vi "CANOpen_SDO Update status channels Dyn Read.vi"(8 "error in (no error)":errorcluster, 9 "Status Data":T2, 10 "Chan Refs":T1[](array[typedef]) format="%.0x", 11 "index of element":i32) -> (0 "error out":errorcluster)   [LabVIEW 2013, in "CANOpen Addon Custom Device.lvlib"]
uses:
  CANOpen Addon Custom Device.lvlib
  Async VIs/CANOpen_Main/SubVIs/CanOpen_SDO Dynamic queue.ctl
  Shared Code/CANOpen_SDO queue W data.ctl
  Shared Code/CANOpen_SDO queue mode.ctl
  Shared Code/CANOpen_PDO Data Type in queue.ctl
  <vilib>/NI Veristand/Custom Device API/Data Reference.ctl
  <vilib>/NI Veristand/Custom Device API/Global Data Refs.vi
  <vilib>/NI Veristand/Custom Device API/Custom Device API.lvlib
  Debug/SubVIs/Global debug.vi
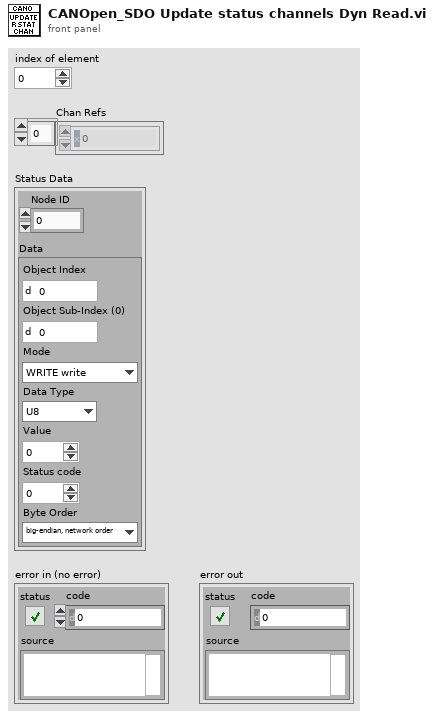
[diagram p1: front panel]
types:
  T1 = typedef "Custom Device API.lvlib/Data Reference.ctl" = i32
  T2 = typedef "CANOpen Addon Custom Device.lvlib/CanOpen_SDO Dynamic queue.ctl" = cluster{"Node ID":u8, "Data":T3}
  T3 = typedef "CANOpen Addon Custom Device.lvlib/CANOpen_SDO queue W data.ctl" = cluster{"Object Index":u16, "Object Sub-Index (0)":u8, "Mode":T4, "Data Type":T5, "Value":dbl, "Status code":dbl, "Byte Order":enum16{"big-endian, network order", "little-endian"}}
  T4 = typedef "CANOpen Addon Custom Device.lvlib/CANOpen_SDO queue mode.ctl" = enum16{"WRITE write", "WRITE response", "READ write", "READ response"}
  T5 = typedef "CANOpen Addon Custom Device.lvlib/CANOpen_PDO Data Type in queue.ctl" = enum16{"U8", "U16", "U32", "I8", "I16", "I32", "Single", "Double"}
  T6 = enum16{"big-endian, network order", "little-endian"}
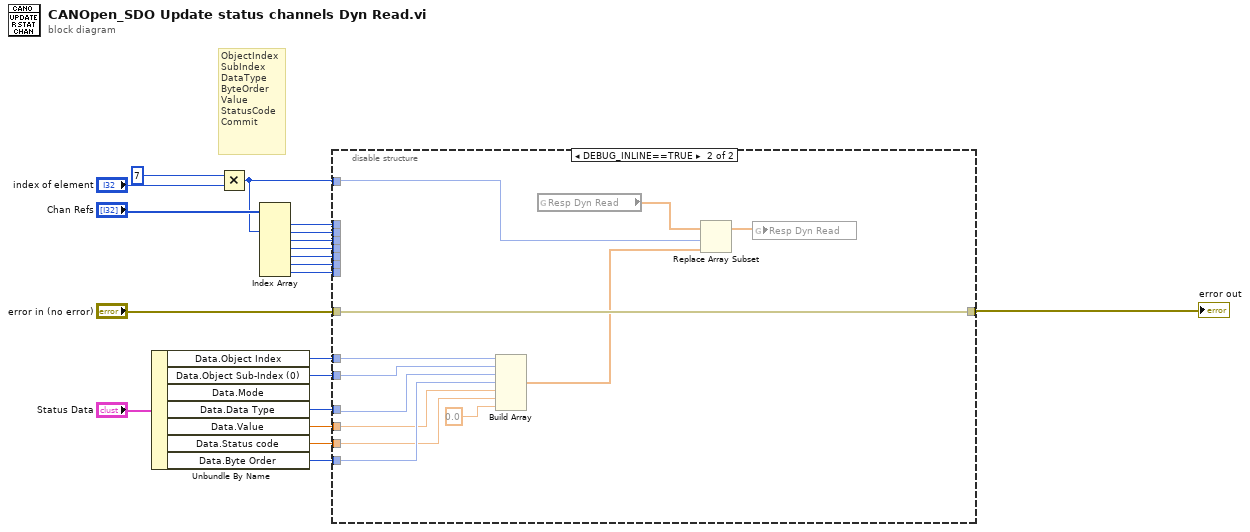
[diagram p0: block diagram]
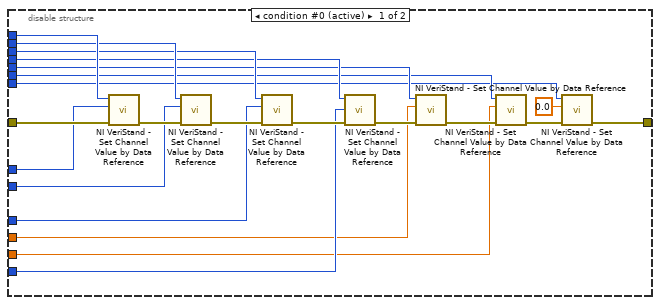
[diagram p2: hidden frame]
diagram:
  # "ObjectIndex\nSubIndex\nDataType\nByteOrder\nValue\nStatusCode\nCommit"
  n1 = Unbundle By Name("Status Data") -> ("Data.Object Index"=w7:u16, "Data.Object Sub-Index (0)"=w6:u8, "Data.Data Type"=w5:T5, "Data.Value"=w3:dbl, "Data.Status code"=w2:dbl, "Data.Byte Order"=w4:T6)  [unwired: 1 out]
  n2 = Multiply(x=7, y="index of element") -> (x*y=w1:i32)
  n3 = Index Array(array="Chan Refs", index #1=w1) -> (element #1=w14:T1, element #2=w13:T1, element #3=w12:T1, element #4=w11:T1, element #5=w10:T1, element #6=w9:T1, element #7=w8:T1)  [unwired: 6 in]
  n4 = disable-structure shown="DEBUG_INLINE==TRUE" {
    disable-tunnel: "error in (no error)" -> [w42 w54]
    disable-tunnel: [w35 w54] -> w20
    disable-tunnel: w14 -> [w34 _]
    disable-tunnel: w13 -> [w33 _]
    disable-tunnel: w12 -> [w32 _]
    disable-tunnel: w11 -> [w31 _]
    disable-tunnel: w10 -> [w30 _]
    disable-tunnel: w9 -> [w29 _]
    disable-tunnel: w8 -> [w28 _]
    disable-tunnel: w7 -> [w27 w53]
    disable-tunnel: w6 -> [w26 w52]
    disable-tunnel: w5 -> [w25 w51]
    disable-tunnel: w4 -> [w24 w46]
    disable-tunnel: w3 -> [w23 w45]
    disable-tunnel: w2 -> [w22 w44]
    disable-tunnel: w1 -> [_ w50]
    frame condition #0 (active) {
      n5 = call <vilib>:"NI VeriStand - Set Channel Value by Data Reference.vi"("error in (no error)"=w42, "Value"=w27, "Data Reference in"=w34) -> ("error out"=w41:errorcluster)  [unwired: 8 in]
      n6 = call <vilib>:"NI VeriStand - Set Channel Value by Data Reference.vi"("error in (no error)"=w41, "Value"=w26, "Data Reference in"=w33) -> ("error out"=w40:errorcluster)  [unwired: 8 in]
      n7 = call <vilib>:"NI VeriStand - Set Channel Value by Data Reference.vi"("error in (no error)"=w40, "Value"=w25, "Data Reference in"=w32) -> ("error out"=w39:errorcluster)  [unwired: 8 in]
      n8 = call <vilib>:"NI VeriStand - Set Channel Value by Data Reference.vi"("error in (no error)"=w39, "Value"=w24, "Data Reference in"=w31) -> ("error out"=w38:errorcluster)  [unwired: 8 in]
      n9 = call <vilib>:"NI VeriStand - Set Channel Value by Data Reference.vi"("error in (no error)"=w38, "Value"=w23, "Data Reference in"=w30) -> ("error out"=w37:errorcluster)  [unwired: 8 in]
      n10 = call <vilib>:"NI VeriStand - Set Channel Value by Data Reference.vi"("error in (no error)"=w37, "Value"=w22, "Data Reference in"=w29) -> ("error out"=w36:errorcluster)  [unwired: 8 in]
      n11 = call <vilib>:"NI VeriStand - Set Channel Value by Data Reference.vi"("error in (no error)"=w36, "Value"=0.0, "Data Reference in"=w28) -> ("error out"=w35:errorcluster)  [unwired: 8 in]
    }
    frame condition #1 {
      n12 = Build Array(w53, w52, w51, w46, w45, w44, 0.0 ("element")) -> (w48:dbl[])
      n13 = global read "Global debug.vi" "Resp Dyn Read"() -> (w49:dbl[])
      n14 = Replace Array Subset(array=w49, new element=w48, index=w50) -> (w47:dbl[])
      n15 = global write "Global debug.vi" "Resp Dyn Read"(w47) -> ()
    }
  }
  "error out" <- w20
